vi "未命名 1.vi"() -> ()   [LabVIEW 2017]
panel:
  out "Y":dbl
  in  "b":dbl
  in  "X":dbl
  in  "K":dbl
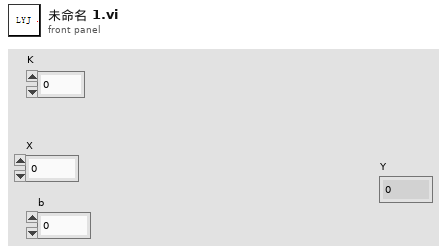
[diagram p1: front panel]
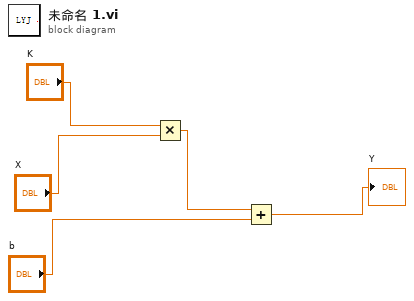
[diagram p0: block diagram]
diagram:
  n1 = Multiply(x="K", y="X") -> (x*y=w2:dbl)
  n2 = Add(x=w2, y="b") -> (x+y=→"Y":dbl)
